vi "1-Tap 10-Bit Camera with Frame Trigger (FPGA).vi"() -> ()   [LabVIEW 2012]
doc: "This is the FPGA VI for the 1-Tap 10-Bit Camera with Frame Trigger example. This example demonstrates how to acquire images from a 1-tap, 10-bit Base Camera Link camera connected to the NI 1483 and transfer the images to the host via a DMA FIFO. This example supports area scan and line scan cameras for both continuous and finite acquisitions.\n\nThis example also demonstrates the generation of a camera trigger using the Camera Control 1 signal on the Camera Link cable. The pulse width of this trigger can be customized to control the exposure of the camera, if supported. The source of the trigger can be a rising edge signal from the host VI or a rising edge on the TTL In 0 signal.\n\nAdditionally, the example demonstrates the serial server, which allows third-party camera configuration utilities to communicate with the camera using the Camera Link serial interface while this VI is running."
uses:
  Common/CL Signal Mapping.ctl
  Common/CL Configuration.ctl
  <vilib>/Platform/TimedLoop/XDataNode/timing_clust.ctl
  <vilib>/Platform/TimedLoop/XDataNode/nitl_modes.ctl
  <vilib>/Platform/TimedLoop/XDataNode/wakeup.ctl
  <vilib>/rvi/eio/common/nirviEmuTemplateMethod_errors.vi
  <vilib>/rvi/Emulation/niFpgaSctlEmulationRegisterWithScheduler.vi
  <vilib>/rvi/Emulation/niFpgaSctlEmulationScheduler.vi
  Common/CL Data to Pixels/1 Tap 10-Bit.vi
  <vilib>/rvi/interface/RandomDataEmulation/nirviRandomDataFPGAFIFO.vi
  <vilib>/rvi/interface/RandomDataEmulation/niFpgaRandomDataHandleErrors.vi
  <vilib>/rvi/Emulation/niFpgaSctlEmulationGlobalWrite.vi
  <vilib>/Platform/TimedLoop/XDataNode/XDataNode.xnode
  <vilib>/eio/EIONode/EIONode.xnode
  <vilib>/rvi/DataTransferAndStorage/Container/XNode/niFpgaContainer.xnode
  <vilib>/rvi/interface/RandomDataEmulation/nirviRandomDataFpgaReadWriteTemplate.vi
  <vilib>/Platform/TimedLoop/XDataNode/XDNodeRunTimeDep.lvlib
panel:
  in  "CL Config.Configuration":T1
  in  "CL Config.Signal Mapping":T2
  in  "CL Config.Line Scan":bool
  in  "CL Config.DVAL Active High":bool=TRUE
  in  "CL Config.LVAL Active High":bool=TRUE
  in  "CL Config.FVAL Active High":bool=TRUE
  in  "CL Config.Spare Active High":bool=TRUE
  in  "Acq Control.Line Scan Height":u32
  in  "Acq Control.Frames To Acq":u32
  in  "Acq Control.Acquire":bool
  in  "Acq Control.Cancel Acq":bool
  in  "Acq Control.Ignore DVAL":bool
  in  "Acq Control.Initialize":bool
  out "Acq Status.Acq In Progress":bool
  out "Acq Status.Clocks Per Line":u32
  out "Acq Status.Frames Acq'd":u32
  out "Acq Status.Lines Per Frame":u32
  out "Acq Status.DMA Write Timeout":bool
  out "Acq Status.Initialized":bool
  in  "UART.Baud Rate":u8
  in  "UART.Transmit":bool
  in  "UART.Tx Data":u8[](array[numeric])=[0, 0, 0, 0, 0, 0, 0, 0, 0, 0] format="%02x"
  in  "UART.Set Baud Rate":bool
  in  "UART.Byte Mode":bool=TRUE
  out "UART.Rx Ready":bool
  out "UART.Break Indicator":bool
  out "UART.Framing Error":bool
  out "UART.Overrun Error":bool
  out "UART.Tx Ready":bool
  out "UART.Rx Data":u8 format="%02x"
  in  "UART.Receive":bool
  in  "Trigger.Trigger Pulse Width (40 MHz Ticks)":u32=4000
  in  "Trigger.Send Software Trigger":bool
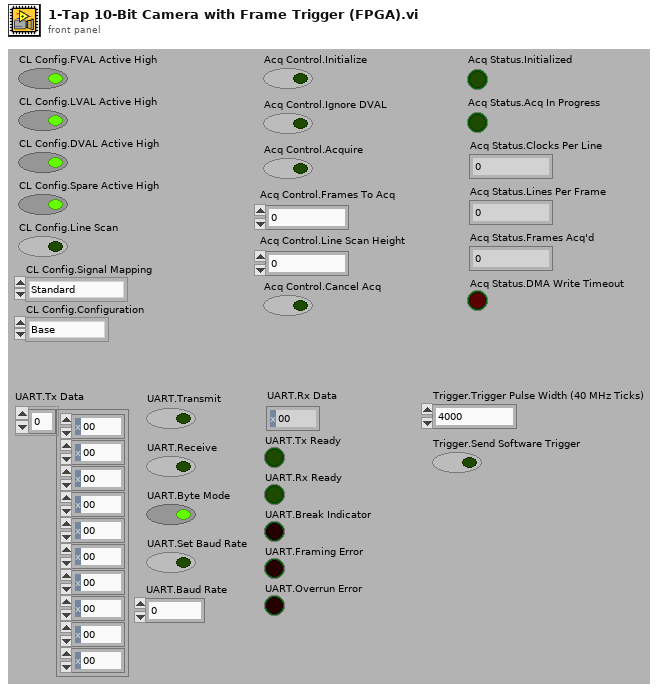
[diagram p1: front panel]
types:
  T1 = typedef "CL Configuration.ctl" = enum8{"Base", "Medium", "Full"}
  T2 = typedef "CL Signal Mapping.ctl" = enum8{"Standard", "Basler 10-tap", "Vosskühler 10-tap"}
  T3 = typedef "XDNodeRunTimeDep.lvlib/timing_clust.ctl" = cluster{"Expected End [f-1]":u64, "Actual End [f-1]":u64, "Finished Late? [f-1]":bool, "Expected End [i-1]":u64, "Actual End [i-1]":u64, "Finished Late? [i-1]":bool, "Expected Start [i]":u64, "Actual Start [i]":u64, "Expected Start [f]":u64, "Actual Start [f]":u64, "Source Name":string, "Structure Name":string, "Period":i64, "Deadline":i64, "Offset":i64, "Start":i64, "Priority":i32, "Timeout":i32, "Mode":T4, "Wakeup Reason":T5, "Error":errorcluster, "Source Type":string, "Secondary Source Type":string, "Global End Time":u64, "Global Start Time":u64, "Frame Duration":u64, "Iteration Duration":u64, "Assigned CPU":i32, "I/O Scan Engine Mode":u32}
  T4 = typedef "XDNodeRunTimeDep.lvlib/nitl_modes.ctl" = enum32{"No Change", "Process missed periods, maintain original phase", "Discard missed periods, maintain original phase", "Process missed periods, ignore original phase", "Discard missed periods, ignore original phase"}
  T5 = typedef "XDNodeRunTimeDep.lvlib/wakeup.ctl" = enum32{"Normal", "Aborted", "Asynchronous wakeup", "Timing source error", "Timed loop error", "Timeout"}
  T6 = cluster{"Enables Valid":bool, "Frame Valid":bool, "Line Valid":bool, "Data Valid":bool}
  T7 = cluster{"Tx Data":u8[], "Transmit":bool, "Receive":bool, "Byte Mode":bool, "Set Baud Rate":bool, "Baud Rate":u8}
  T8 = cluster{"Rx Data":u8, "Turn Off Transmit":bool, "Turn Off Receive":bool, "Turn Off Set Baud Rate":bool, "Tx Ready":bool, "Rx Ready":bool, "Break Indicator":bool, "Framing Error":bool, "Overrun Error":bool}
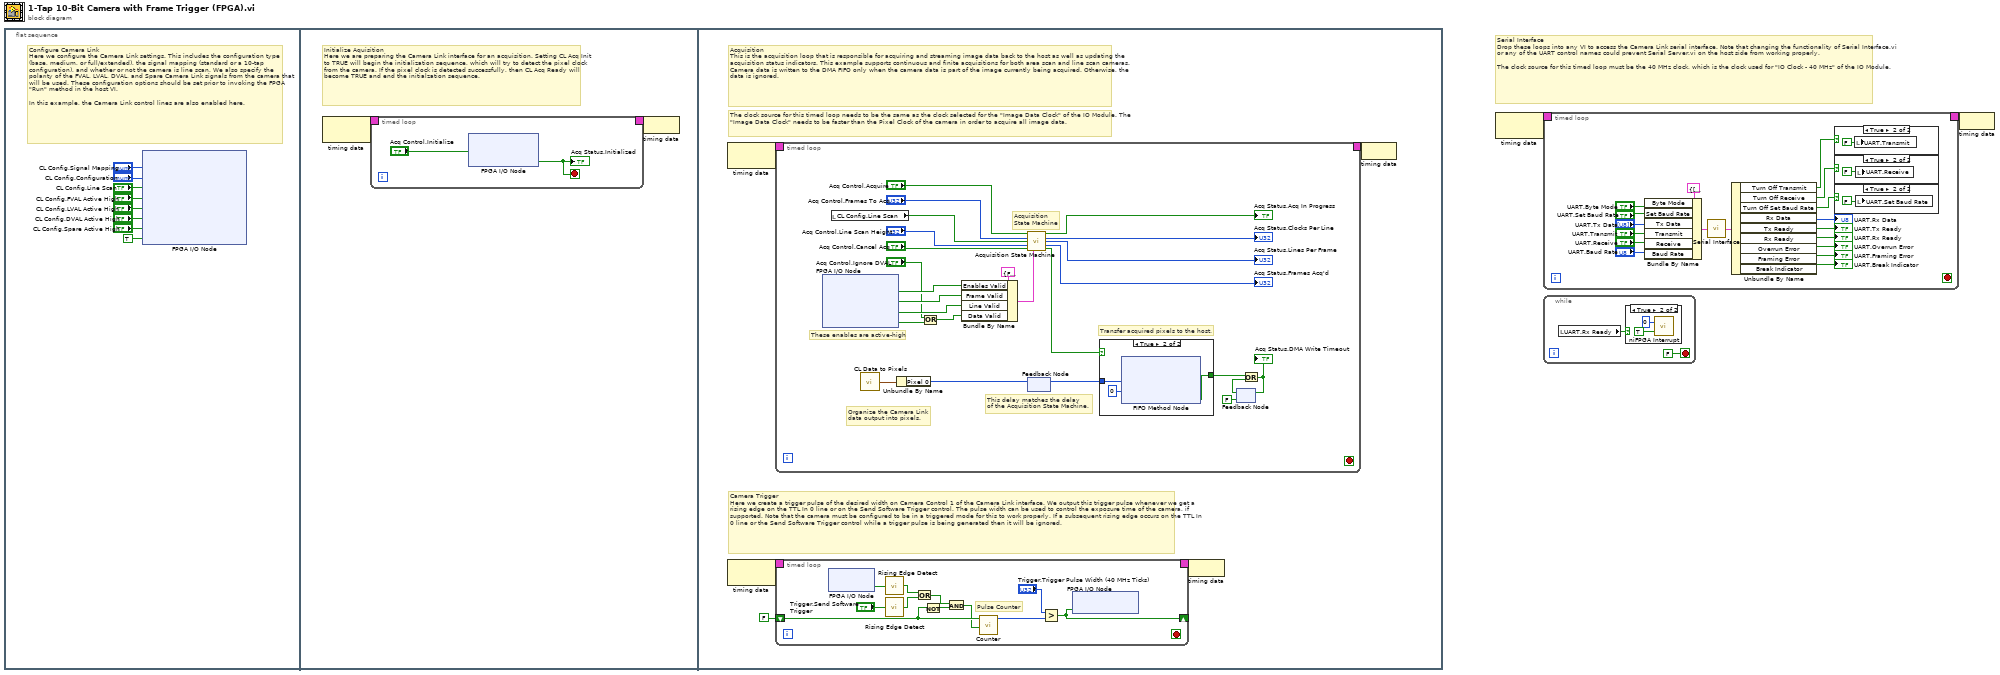
[diagram p0: block diagram]
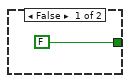
[diagram p6: hidden frame]
diagram:
  # "Serial Interface\nDrop these loops into any VI to access the Camera Link serial interface. Note that changing the functionality of Serial Interface.vi or any of the UART control names could prevent Serial Server.vi on the host side from working properly.\n\nThe clock source for this timed loop must be the 40 MHz clock, which is the clock used for \"IO Clock - 40 MHz\" of the IO Module."
  n1 = flat-sequence {
    frame #0 {
      # "Configure Camera Link\nHere we configure the Camera Link settings. This includes the configuration type (base, medium, or full/extended), the signal mapping (standard or a 10-tap configuration), and whether or not the camera is line scan. We also specify the polarity of the FVAL, LVAL, DVAL, and Spare Camera Link signals from the camera that will be used. These configuration options should be set prior to invoking the FPGA \"Run\" method in the host VI.\n\nIn this example, the Camera Link control lines are also enabled here."
      n2 = xnode "FPGA I/O Node"("CL Set Signal Mapping"="CL Config.Signal Mapping", "CL Set Configuration"="CL Config.Configuration", "CL Set Line Scan"="CL Config.Line Scan", "CL Set FVAL Active High"="CL Config.FVAL Active High", "CL Set LVAL Active High"="CL Config.LVAL Active High", "CL Set DVAL Active High"="CL Config.DVAL Active High", "CL Set Spare Active High"="CL Config.Spare Active High", "CL Control Enable"=TRUE ("IO Module\\CL Control Enable")) -> ()  [unwired: 8 in, 8 out]
    }
    frame #1 {
      # "Initialize Aquisition\nHere we are preparing the Camera Link interface for an acquisition. Setting CL Acq Init to TRUE will begin the initialization sequence, which will try to detect the pixel clock from the camera. If the pixel clock is detected successfully, then CL Acq Ready will become TRUE and end the initialzation sequence."
      n3 = node-c288() -> (w12:T3)  [unwired: 1 out]
      n4 = timed-loop {
        timing: w12 -> [_]
        timing-out: [_] -> w11
        stop <- w13 stop-if-true
        n5 = xnode "FPGA I/O Node"("CL Acq Init"="Acq Control.Initialize") -> ("CL Acq Ready"=w13:bool)  [unwired: 2 in, 2 out]
        "Acq Status.Initialized" <- w13
      }
      n6 = node-c288(w11) -> ()
    }
    frame #2 {
      # "The clock source for this timed loop needs to be the same as the clock selected for the \"Image Data Clock\" of the IO Module. The \"Image Data Clock\" needs to be faster than the Pixel Clock of the camera in order to acquire all image data."
      # "Acquisition\nThis is the acquisition loop that is responsible for acquiring and streaming image data back to the host as well as updating the acquisition status indicators. This example supports continuous and finite acquisitions for both area scan and line scan cameras. Camera data is written to the DMA FIFO only when the camera data is part of the image currently being acquired. Otherwise, the data is ignored."
      # "Camera Trigger\nHere we create a trigger pulse of the desired width on Camera Control 1 of the Camera Link interface. We output this trigger pulse whenever we get a rising edge on the TTL In 0 line or on the Send Software Trigger control. The pulse width can be used to control the exposure time of the camera, if supported. Note that the camera must be configured to be in a triggered mode for this to work properly. If a subsequent rising edge occurs on the TTL In 0 line or the Send Software Trigger control while a trigger pulse is being generated then it will be ignored."
      n7 = node-c288() -> (w23:T3)  [unwired: 1 in]
      n8 = node-c288() -> (w21:T3)  [unwired: 1 in]
      n9 = timed-loop {
        timing: w23 -> [_]
        timing-out: [_] -> w22
        stop <- _ stop-if-true
        # "Transfer acquired pixels to the host."
        # "Organize the Camera Link\ndata output into pixels."
        # "These enables are active-high"
        # "This delay matches the delay\nof the Acquisition State Machine."
        # "Acquisition\nState Machine"
        n10 = xnode "FPGA I/O Node"() -> ("CL Output Valid"=w48:bool, "CL Frame Valid"=w47:bool, "CL Line Valid"=w46:bool, "CL Data Valid"=w43:bool)  [unwired: 4 in, 4 out]
        n11 = local read "CL Config.Line Scan"() -> (w40:bool)
        n12 = call-poly "CL Data to Pixels.vi"() -> ("Pixels"=w63:cluster{"Pixel 0":u16})  [unwired: 1 in]
        n13 = Unbundle By Name(w63) -> ("Pixel 0"=w62:u16)
        n14 = Or(x="Acq Control.Ignore DVAL", y=w43) -> (x .or. y?=w42:bool)
        n15 = Bundle By Name(cluster=T6 {"Enables Valid"=FALSE, "Frame Valid"=FALSE, "Line Valid"=FALSE, "Data Valid"=FALSE} ("Enables"), "Enables Valid"=w48, "Frame Valid"=w47, "Line Valid"=w46, "Data Valid"=w42) -> (w45:T6)
        n16 = call "Acquisition State Machine.vi"("Acquire"="Acq Control.Acquire", "Frames to Acquire"="Acq Control.Frames To Acq", "Line Scan"=w40, "Line Scan Height"="Acq Control.Line Scan Height", "Cancel Acq"="Acq Control.Cancel Acq", "Enables"=w45) -> ("Acq In Progress"=→"Acq Status.Acq In Progress":bool, "Num Clocks Per Line"=→"Acq Status.Clocks Per Line":u32, "Num Lines Per Frame"=→"Acq Status.Lines Per Frame":u32, "Num Frames Acq'd"=→"Acq Status.Frames Acq'd":u32, "Capture Cycle"=w60:bool)  [unwired: 4 in, 1 out]
        n17 = feedback-in #1(w62) -> ()
        n18 = feedback #1() -> (w61:u16)  [unwired: 1 in]
        n19 = case shown="True" w60 {
          tunnel: [FALSE ("Timed Out?") w65] -> w58
          tunnel: w61 -> [_ w66]
          frame False {
          }
          frame True {
            n20 = xnode ("FIFO Method Node")("Element"=w66, "Timeout"=0) -> ("Timed Out?"=w65:bool)  [unwired: 1 in, 1 out]
          }
        }
        n21 = feedback #2(FALSE) -> (w57:bool)
        n22 = Or(x=w58, y=w57) -> (x .or. y?=w56:bool)
        "Acq Status.DMA Write Timeout" <- w56
        n23 = feedback-in #2(w56) -> ()
      }
      n24 = timed-loop {
        timing: w21 -> [_]
        timing-out: [_] -> w20
        shift-right: [w32] -> _
        shift-left: FALSE -> [w29]
        stop <- _ stop-if-true
        # "Pulse Counter"
        n25 = xnode "FPGA I/O Node"() -> ("TTL 0"=w27:bool)  [unwired: 1 in, 1 out]
        n26 = call "Rising Edge Detect.vi"("Input"=w27) -> ("Pulse"=w26:bool)  [unwired: 4 in]
        n27 = call "Rising Edge Detect.vi"("Input"="Trigger.Send Software Trigger") -> ("Pulse"=w24:bool)  [unwired: 4 in]
        n28 = Or(x=w26, y=w24) -> (x .or. y?=w31:bool)
        n29 = Not(x=w29) -> (.not. x?=w30:bool)
        n30 = And(x=w31, y=w30) -> (x .and. y?=w28:bool)
        n31 = call "Counter.vi"("Restart?"=w28, "Increment?"=w29) -> ("Count"=w33:u32)  [unwired: 9 in]
        n32 = Greater?(x="Trigger.Trigger Pulse Width (40 MHz Ticks)", y=w33) -> (0:w32:bool)
        n33 = xnode "FPGA I/O Node"("CL Control 1"=w32) -> ()  [unwired: 1 in, 1 out]
      }
      n34 = node-c288(w20) -> ()
      n35 = node-c288(w22) -> ()
    }
  }
  n36 = node-c288() -> (w2:T3)  [unwired: 1 out]
  n37 = timed-loop {
    timing: w2 -> [_]
    timing-out: [_] -> w1
    stop <- _ stop-if-true
    n38 = Bundle By Name(cluster=T7 {"Tx Data"=[0, 0, 0, 0, 0, 0, 0, 0, 0, 0], "Transmit"=FALSE, "Receive"=FALSE, "Byte Mode"=TRUE, "Set Baud Rate"=FALSE, "Baud Rate"=0} ("UART Inputs"), "Byte Mode"="UART.Byte Mode", "Set Baud Rate"="UART.Set Baud Rate", "Tx Data"="UART.Tx Data", "Transmit"="UART.Transmit", "Receive"="UART.Receive", "Baud Rate"="UART.Baud Rate") -> (w72:T7)
    n39 = call "Serial Interface.vi"("UART Inputs"=w72) -> ("UART Outputs"=w84:T8)
    n40 = Unbundle By Name(w84) -> ("Turn Off Transmit"=w77:bool, "Turn Off Receive"=w78:bool, "Turn Off Set Baud Rate"=w74:bool, "Rx Data"=→"UART.Rx Data":u8, "Tx Ready"=→"UART.Tx Ready":bool, "Rx Ready"=→"UART.Rx Ready":bool, "Overrun Error"=→"UART.Overrun Error":bool, "Framing Error"=→"UART.Framing Error":bool, "Break Indicator"=→"UART.Break Indicator":bool)
    n41 = case shown="True" w77 {
      frame False {
      }
      frame True {
        n42 = local write "UART.Transmit"(FALSE ("UART.Transmit")) -> ()
      }
    }
    n43 = case shown="True" w78 {
      frame False {
      }
      frame True {
        n44 = local write "UART.Receive"(FALSE ("UART.Receive")) -> ()
      }
    }
    n45 = case shown="True" w74 {
      frame False {
      }
      frame True {
        n46 = local write "UART.Set Baud Rate"(FALSE ("UART.Receive")) -> ()
      }
    }
  }
  n47 = while {
    stop <- FALSE stop-if-true
    n48 = local read "UART.Rx Ready"() -> (w96:bool)
    n49 = case shown="True" w96 {
      frame False {
      }
      frame True {
        n50 = call <vilib>:"niFPGA Interrupt.vi"("Wait Until Cleared (F)"=TRUE ("Wait Until Cleared"), "IRQ Number (0)"=u8 0 ("IRQ Number")) -> ()  [unwired: 1 in]
      }
    }
  }
  n51 = node-c288(w1) -> ()
